vi "Get Device.vi"(8 "error in (no error)":errorcluster, 11 "DeviceDetailPanel in":refnum<class "DeviceDetailPanel.lvclass">) -> (0 "error out":errorcluster, 2 "Device":refnum<class "Device.lvclass">, 3 "DeviceDetailPanel out":refnum<class "DeviceDetailPanel.lvclass">)   [LabVIEW 2020, in "PicoG-App.lvlib" / "DeviceDetailPanel.lvclass"]
uses:
  DeviceDetailPanel.lvclass
  Device/Device.lvclass
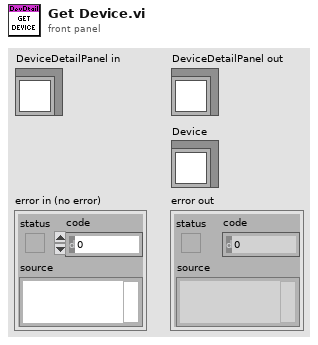
[diagram p1: front panel]
types:
  T1 = typedef "PicoG-App.lvlib/DeviceDetailPanel.lvclass/Ref Data.ctl" = cluster{"Device":refnum<class "Device.lvclass">}
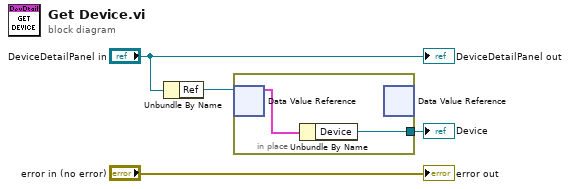
[diagram p0: block diagram]
diagram:
  n1 = Unbundle By Name("DeviceDetailPanel in") -> ("Ref"=w3:refnum<data-value>)
  n2 = in-place {
    in-place-border: [w5] -> w1
    n3 = in-place-dvr #1(w3) -> (w6:T1)  [unwired: 1 out]
    n4 = Unbundle By Name(w6) -> ("Device"=w5:refnum<class "Device.lvclass">)
    n5 = in-place-dvr #1() -> ()  [unwired: 1 in, 2 out]
  }
  "Device" <- w1
  "error out" <- "error in (no error)"
  "DeviceDetailPanel out" <- "DeviceDetailPanel in"
